vi "UTILITY Find File In Folder.vi"(8 "Error In":errorcluster, 10 "File Name":string="RmPid8Stall.lup", 11 "Path":path) -> (0 "Error Out":errorcluster, 3 "appended path":path)   [LabVIEW 2016]
panel:
  out "filenames":string[](array[string])
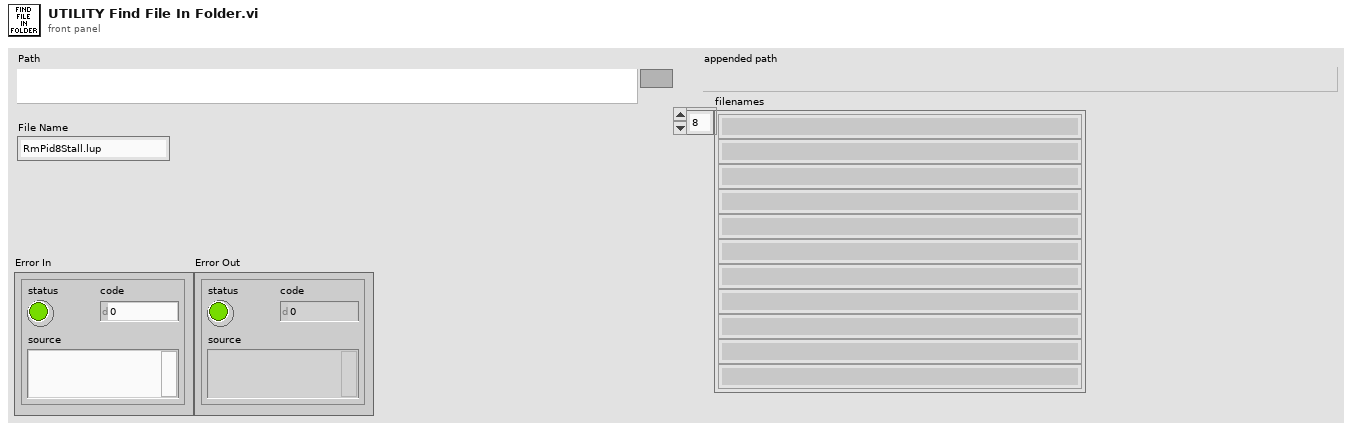
[diagram p1: front panel]
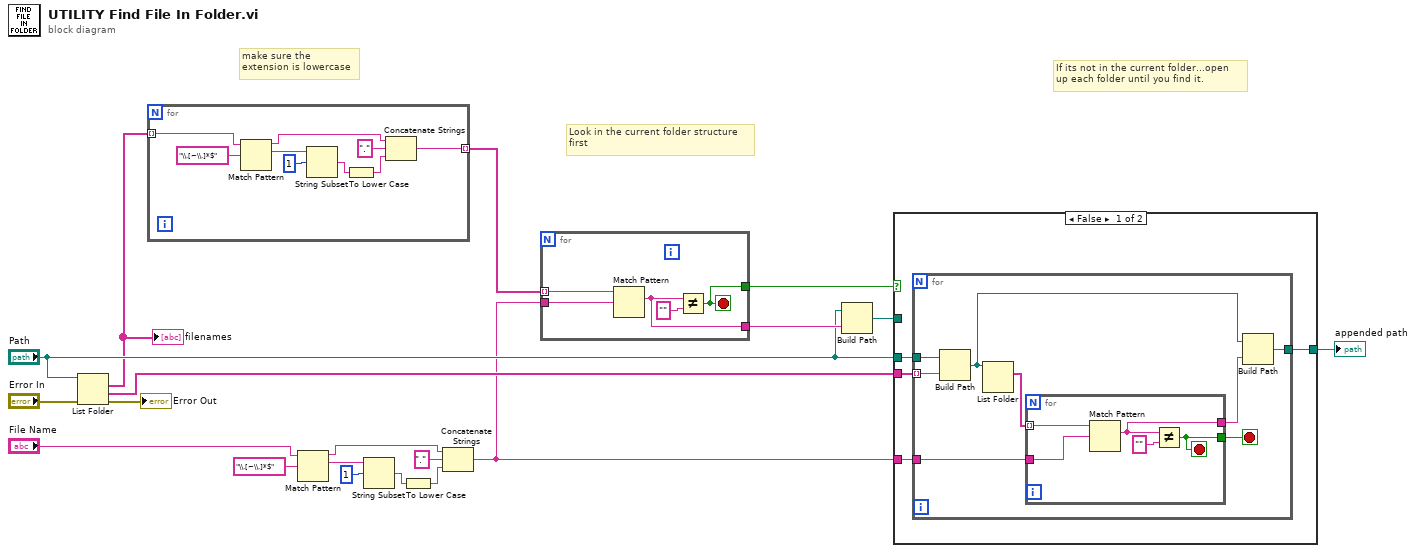
[diagram p0: block diagram]
diagram:
  # "make sure the \nextension is lowercase"
  # "If its not in the current folder...open \nup each folder until you find it."
  # "Look in the current folder structure\nfirst"
  n1 = List Folder(path="Path", error in="Error In") -> (filenames=w2:string[], folder names=w18:string[], error out=→"Error Out":errorcluster)  [unwired: 2 in, 1 out]
  "filenames" <- w2
  n2 = for {
    tunnel: w2 -> [w21] mode=indexing
    tunnel: [w20] -> w1 mode=indexing
    n3 = Match Pattern(string=w21, regular expression="\\.[~\\.]*$") -> (before substring=w26:string, match substring=w24:string)  [unwired: 3 out]
    n4 = String Subset(string=w24, offset (0)=1) -> (substring=w22:string)  [unwired: 1 out]
    n5 = To Lower Case(string=w22) -> (all lower case string=w27:string)
    n6 = Concatenate Strings(w26, "." ("string"), w27) -> (w20:string)
  }
  n7 = Match Pattern(string="File Name", regular expression="\\.[~\\.]*$") -> (before substring=w6:string, match substring=w9:string)  [unwired: 3 out]
  n8 = String Subset(string=w9, offset (0)=1) -> (substring=w11:string)  [unwired: 1 out]
  n9 = To Lower Case(string=w11) -> (all lower case string=w5:string)
  n10 = Concatenate Strings(w6, "." ("string"), w5) -> (w3:string)
  n11 = for {
    tunnel: w1 -> [w33] mode=indexing
    tunnel: [w29] -> w13
    tunnel: [w31] -> w15
    tunnel: w3 -> [w30]
    stop <- w29 stop-if-true
    n12 = Match Pattern(string=w33, regular expression=w30) -> (match substring=w31:string)  [unwired: 1 in, 3 out]
    n13 = Not Equal?(x=w31, y="") -> (x != y?=w29:bool)
  }
  n14 = Build Path(base path="Path", name or relative path=w15) -> (appended path=w12:path)
  n15 = case shown="False" w13 {
    tunnel: [w37 w51] -> w19
    tunnel: w18 -> [w36 _]
    tunnel: w3 -> [w35 _]
    tunnel: "Path" -> [w34 _]
    tunnel: w12 -> [_ w51]
    frame False {
      n16 = for {
        tunnel: w36 -> [w45] mode=indexing
        tunnel: w34 -> [w44]
        tunnel: [w39] -> w37
        tunnel: w35 -> [w38]
        stop <- w42 stop-if-true
        n17 = Build Path(base path=w44, name or relative path=w45) -> (appended path=w40:path)
        n18 = List Folder(path=w40) -> (filenames=w43:string[])  [unwired: 3 in, 3 out]
        n19 = for {
          tunnel: w43 -> [w50] mode=indexing
          tunnel: [w48] -> w42
          tunnel: [w47] -> w41
          tunnel: w38 -> [w46]
          stop <- w48 stop-if-true
          n20 = Match Pattern(string=w50, regular expression=w46) -> (match substring=w47:string)  [unwired: 1 in, 3 out]
          n21 = Not Equal?(x=w47, y="") -> (x != y?=w48:bool)
        }
        n22 = Build Path(base path=w40, name or relative path=w41) -> (appended path=w39:path)
      }
    }
    frame True {
    }
  }
  "appended path" <- w19
